vi "GetDVR.vi"(8 "error in":errorcluster, 11 "OperationRun":refnum<class "OperationRun.lvclass">) -> (0 "error out":errorcluster, 3 "DVRReference":refnum<data-value>)   [LabVIEW 2021, in "ProligentXMLGenerator.lvlib" / "OperationRun.lvclass"]
uses:
  OperationRun.lvclass
  OperationRun.lvclass/OperationRun.ctl
  Base/DateTime/DateTime.lvclass
  Base/ProcessFullName/ProcessFullName.lvclass
  Base/NonEmptyString_65/NonEmptyString_65.lvclass
  Base/ExecutionStatus/ExecutionStatus.lvclass
  Data.ctl
  Base/NonEmptyString_255/NonEmptyString_255.lvclass
  SequenceRun/SequenceRun/SequenceRun.lvclass
  Base/Guid/Guid.lvclass
  Base/FullName/FullName.lvclass
  Base/NonEmptyString_64/NonEmptyString_64.lvclass
  Model/CustomData/CustomData.lvclass
  SequenceRun/SequenceRunReference/SequenceRunReference.lvclass
  Failure/FailureReference/FailureReference.lvclass
  Model/Document/Document.lvclass
  Model/Characteristic/Characteristic.lvclass
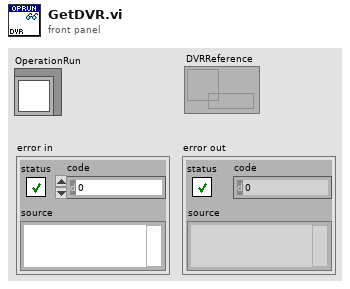
[diagram p1: front panel]
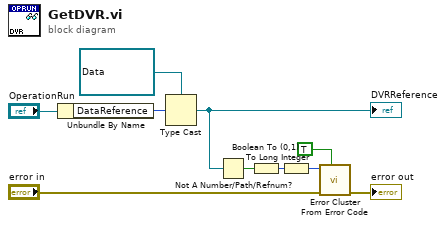
[diagram p0: block diagram]
diagram:
  n1 = Unbundle By Name("OperationRun") -> ("DataReference"=w10:u64)
  n2 = Type Cast(type=refnum<data-value> refnum ("data value reference"), x=w10) -> (*(type *) &x=w6:refnum<data-value>)
  "DVRReference" <- w6
  n3 = Not A Number/Path/Refnum?(number/path/refnum=w6) -> (NaN/Path/Refnum?=w3:bool)
  n4 = Boolean To (0,1)(Boolean=w3) -> (0, 1=w4:i16)
  n5 = To Long Integer(number=w4) -> (32bit integer=w2:i32)
  n6 = call <vilib>:"Error Cluster From Error Code.vi"("show call chain? (False)"=TRUE, "error in (no error)"="error in", "error code (0)"=w2) -> ("error out"=→"error out":errorcluster)  [unwired: 6 in]
